vi "Plot DATA.vi"(1 "Ch 5":dbl[](array[numeric])=[0.0, 0.0, 0.0, 0.0, 0.0, 0.0, 0.0, 0.0, 0.0, 0.0, 0.0, 0.0], 2 "Ch 4":dbl[](array[numeric])=[0.0, 0.0, 0.0, 0.0, 0.0, 0.0, 0.0, 0.0, 0.0, 0.0, 0.0, 0.0], 3 "Ch 2":dbl[](array[numeric])=[0.0, 0.0, 0.0, 0.0, 0.0, 0.0, 0.0, 0.0, 0.0, 0.0, 0.0, 0.0], 4 "Ch 6":dbl[](array[numeric])=[0.0, 0.0, 0.0, 0.0, 0.0, 0.0, 0.0, 0.0, 0.0, 0.0, 0.0, 0.0], 5 "Ch 3":dbl[](array[numeric])=[0.0, 0.0, 0.0, 0.0, 0.0, 0.0, 0.0, 0.0, 0.0, 0.0, 0.0, 0.0], 6 "Ch 1":dbl[](array[numeric])=[0.0, 0.0, 0.0, 0.0, 0.0, 0.0, 0.0, 0.0, 0.0, 0.0, 0.0, 0.0], 7 "Current time":timestamp[](array[timestamp])) -> (0 "Graph Out":T1(array[cluster]))   [LabVIEW 2018]
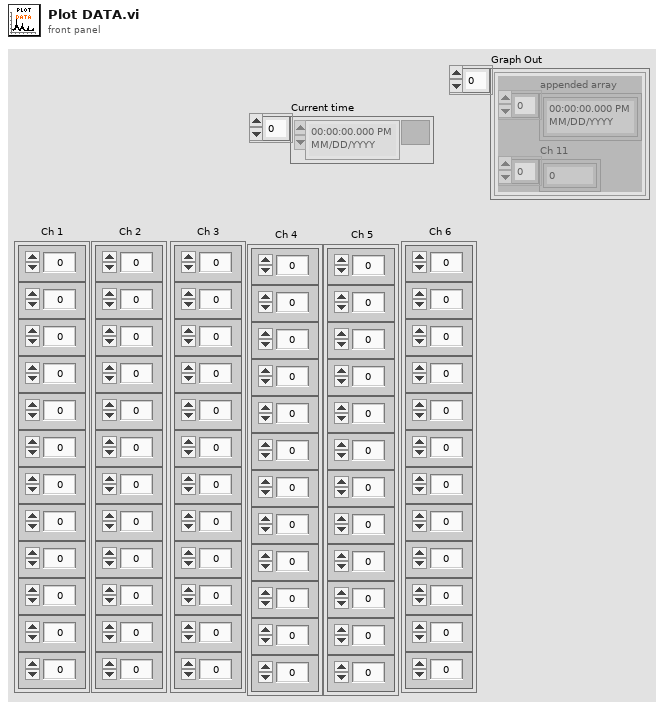
[diagram p1: front panel]
types:
  T1 = cluster{"appended array":timestamp[], "Ch 11":dbl[]}[]
  T2 = cluster{"Current time":timestamp[], "Ch 1":dbl[]}
  T3 = cluster{"Current time":timestamp[], "Ch 2":dbl[]}
  T4 = cluster{"Current time":timestamp[], "Ch 3":dbl[]}
  T5 = cluster{"Current time":timestamp[], "Ch 4":dbl[]}
  T6 = cluster{"Current time":timestamp[], "Ch 5":dbl[]}
  T7 = cluster{"Current time":timestamp[], "Ch 6":dbl[]}
  T8 = cluster{"Current time":timestamp[], "Ch 6":dbl[]}[]
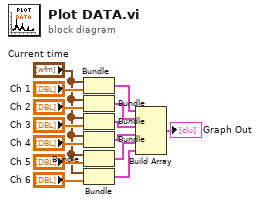
[diagram p0: block diagram]
diagram:
  n1 = Bundle("Current time"="Current time", "Ch 1"="Ch 1") -> (w14:T2)  [unwired: 1 in]
  n2 = Bundle("Current time"="Current time", "Ch 2"="Ch 2") -> (w13:T3)  [unwired: 1 in]
  n3 = Bundle("Current time"="Current time", "Ch 3"="Ch 3") -> (w12:T4)  [unwired: 1 in]
  n4 = Bundle("Current time"="Current time", "Ch 4"="Ch 4") -> (w11:T5)  [unwired: 1 in]
  n5 = Bundle("Current time"="Current time", "Ch 5"="Ch 5") -> (w10:T6)  [unwired: 1 in]
  n6 = Bundle("Current time"="Current time", "Ch 6"="Ch 6") -> (w9:T7)  [unwired: 1 in]
  n7 = Build Array(w14, w13, w12, w11, w10, w9) -> (→"Graph Out":T8)
